vi "scale sequence 0,,1.vi"(10 "Data":dbl[](array[numeric]), 11 "map sequence":dbl[](array[numeric])) -> (0 "offset":dbl, 1 "range":dbl, 3 "Scaled Array":dbl[](array[numeric]))   [LabVIEW 2018]
panel:
  out "Waveform Graph":dbl[](graph)
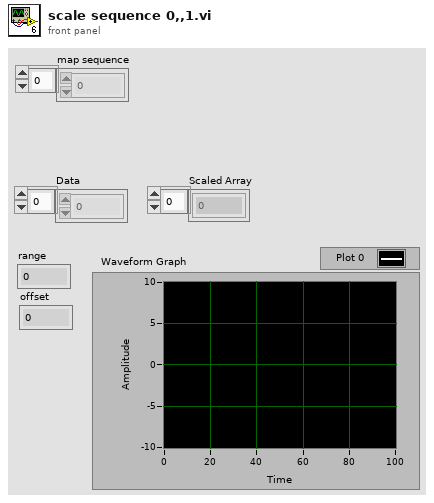
[diagram p1: front panel]
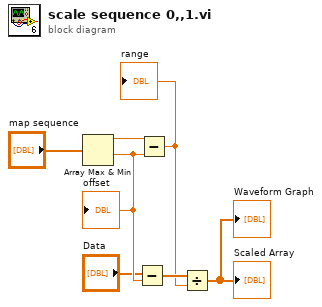
[diagram p0: block diagram]
diagram:
  n1 = Array Max & Min(array="map sequence") -> (max value=w7:dbl, min value=w6:dbl)  [unwired: 2 out]
  "offset" <- w6
  n2 = Subtract(x="Data", y=w6) -> (x-y=w4:dbl[])
  n3 = Subtract(x=w7, y=w6) -> (x-y=w3:dbl)
  "range" <- w3
  n4 = Divide(x=w4, y=w3) -> (x/y=→"Scaled Array" →"Waveform Graph":dbl[])
